vi "User32dllAPI.SetWindowPos.vi"(8 "error in (no error)":errorcluster, 9 "Flags (SHOWWINDOW)":T1=64 items=["NOSIZE"=1, "NOMOVE"=2, "NOZORDER"=4, "NOREDRAW"=8, "NOACTIVATE"=16, "DRAWFRAME"=32, "SHOWWINDOW"=64, "HIDEWINDOW"=128, "NOCOPYBITS"=256, "NOSENDCHANGING"=1024, "DEFERERASE"=8192, "ASYNCWINDOWPOS"=16384], 10 "WinPos":cluster{"X":i32, "Y":i32, "dX":i32, "dY":i32}, 11 "hWnd in":i32) -> (0 "error out":errorcluster, 3 "hWnd out":i32)   [LabVIEW 2019, in "Tools.lvlib"]
uses:
  Tools.lvlib
  User32dllAPI.SetWindowPos.Flag.ctl
  user32.dll
panel:
  in  "User32dllAPI.SetWindowPos.Flag":T1 items=["NOSIZE"=1, "NOMOVE"=2, "NOZORDER"=4, "NOREDRAW"=8, "NOACTIVATE"=16, "DRAWFRAME"=32, "SHOWWINDOW"=64, "HIDEWINDOW"=128, "NOCOPYBITS"=256, "NOSENDCHANGING"=1024, "DEFERERASE"=8192, "ASYNCWINDOWPOS"=16384]
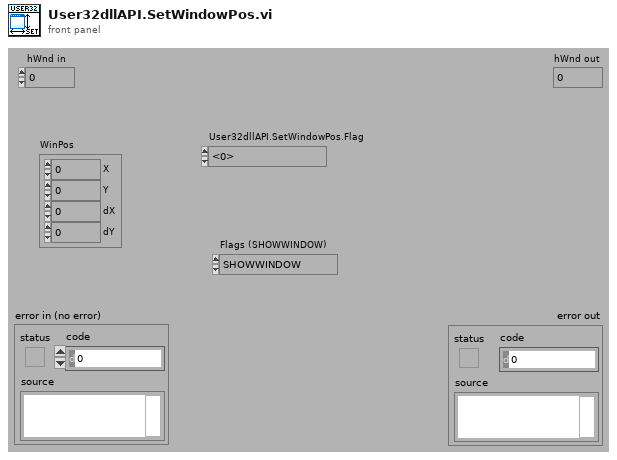
[diagram p1: front panel]
types:
  T1 = typedef "Tools.lvlib/User32dllAPI.SetWindowPos.Flag.ctl" = u32
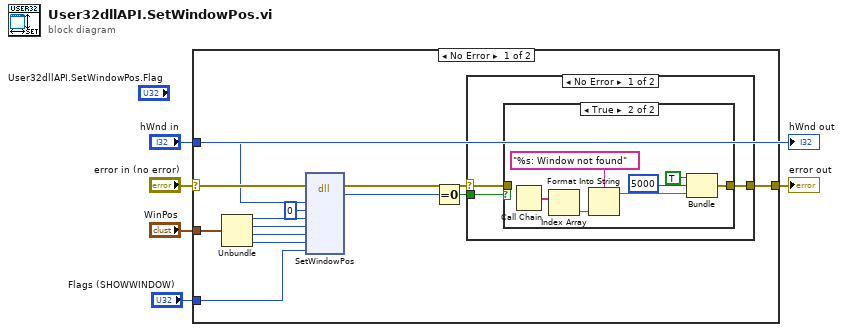
[diagram p0: block diagram]
diagram:
  n1 = case shown="No Error" "error in (no error)" {
    selector: "error in (no error)" -> [w16 w31]
    tunnel: [w17 w31] -> w4
    tunnel: "hWnd in" -> [w6 _]
    tunnel: "WinPos" -> [w13 _]
    tunnel: "Flags (SHOWWINDOW)" -> [w8 _]
    frame No Error {
      n2 = Unbundle(w13) -> ("X"=w12:i32, "Y"=w11:i32, "dX"=w9:i32, "dY"=w10:i32)
      n3 = dll-call lib="USER32.DLL" fn="SetWindowPos"(error in=w16, "hWnd"=w6, "hWndInsertAfter"=0 ("TOP MOST"), "X"=w12, "Y"=w11, "cx"=w9, "cy"=w10, "uFlags"=w8) -> (error out=w7:errorcluster, "bool"=w15:i32)  [unwired: 9 in, 1 out]
      n4 = Equal To 0?(x=w15) -> (x = 0?=w18:bool)
      n5 = case shown="No Error" w7 {
        selector: w7 -> [w19 w30]
        tunnel: w18 -> [w21 _]
        tunnel: [w20 w30] -> w17
        frame No Error {
          n6 = case shown="True" w21 {
            tunnel: [w22 w23] -> w20
            tunnel: w19 -> [w22 _]
            frame False {
            }
            frame True {
              n7 = Call Chain() -> (call chain=w29:string[])
              n8 = Index Array(array=w29) -> (element=w28:string)  [unwired: 1 in]
              n9 = Format Into String(format string="%s: Window not found", w28) -> (resulting string=w26:string)  [unwired: 2 in, 1 out]
              n10 = Bundle("status"=TRUE, "code"=5000, w26) -> (w23:cluster{"status":bool, "code":i32, string})  [unwired: 1 in]
            }
          }
        }
        frame Error {
        }
      }
    }
    frame Error {
    }
  }
  "error out" <- w4
  "hWnd out" <- "hWnd in"
